vi "Sequencer UI - User Event - Inbound&Outbound (Solution).vi"(10 "Outbound User Events":T1, 11 "Inbound User Events":T2) -> ()   [LabVIEW 2019]
uses:
  typedefs/step.data--Cluster.ctl
  typedefs/step.IO.data--Cluster.ctl
  typedefs/IOType--Enum.ctl
  <userlib>/_OpenG.lib/file/file.llb/File Exists - Scalar__ogtk.vi
  <userlib>/_OpenG.lib/file/file.llb/Valid Path - Traditional__ogtk.vi
panel:
  out "timer value":u32
  out "Seq. Aborted?":bool
  out "Seq. Loaded?":bool
  out "Seq. Running?":bool
  out "AO Chart":cluster{"[0]":dbl, "[1]":dbl}(graph)
  out "Running Step ID":string caption="Step ID"
  out "States History":string caption="Last State"
  out "Sequence MCL Ref":i32(listbox) caption="Sequence"
  in  "Abort Sequence":bool
  in  "Run Sequence":bool
  in  "Load Sequence":bool
  in  "Exit":bool
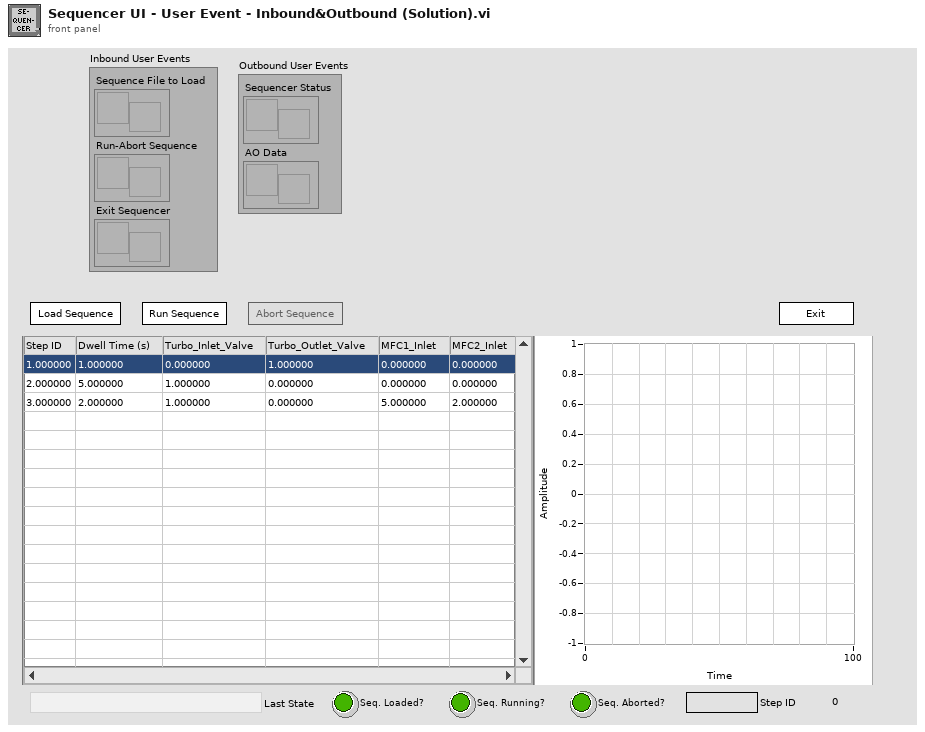
[diagram p1: front panel]
types:
  T1 = cluster{"Sequencer Status":refnum<user-event>, "AO Data":refnum<user-event>}
  T2 = cluster{"Sequence File to Load":refnum<user-event>, "Run-Abort Sequence":refnum<user-event>, "Exit Sequencer":refnum<user-event>}
  T3 = enum32{"invalid app kind", "Development System", "Run Time System", "Student Edition", "Embedded LabVIEW", "Evaluation", "Custom"}
  T4 = enum32{"Invalid", "Standard", "Closed", "Hidden", "Minimized", "Maximized"}
  T5 = enum8{"Enabled", "Disabled", "Disabled and Grayed Out"}
  T6 = typedef "step.data--Cluster.ctl" = cluster{"Step ID":string, "Dwell Time(s)":dbl, "Recipe Step":T7[]}
  T7 = typedef "step.IO.data--Cluster.ctl" = cluster{"IO Name":string, "IO Type":T8, "IO Value":variant}
  T8 = typedef "IOType--Enum.ctl" = enum16{"<Undefined>", "DO", "DI", "AO", "AI"}
  T9 = cluster{"Core":cluster{"Current VI Reference":refnum<vi>, "Close Panel on Exit?":bool}, "Seq. Loaded?":bool, "Sequence file path":path, "Sequence Data [ ]":T6[], "Sequence MCL Ref":refnum<vi>, "DO Data [ ]":cluster{"DO Name":string, "DO Value":variant}[], "AO Data [ ]":cluster{"AO Name":string, "AO Value":variant}[], "Running Step #":i32, "Seq. Running?":bool, "Seq. Aborted?":bool, "Inbound User Events":cluster{"Sequence File to Load":refnum<user-event>, "Run-Abort Sequence":refnum<user-event>, "Exit Sequencer":refnum<user-event>}, "Outbound User Events":cluster{"Sequencer Status":refnum<user-event>, "AO Data":refnum<user-event>}}
  T10 = cluster{"Current VI Reference":refnum<vi>, "Close Panel on Exit?":bool}
  T11 = cluster{"Seq. Loaded?":bool, "Seq. Running?":bool, "Seq. Aborted?":bool}
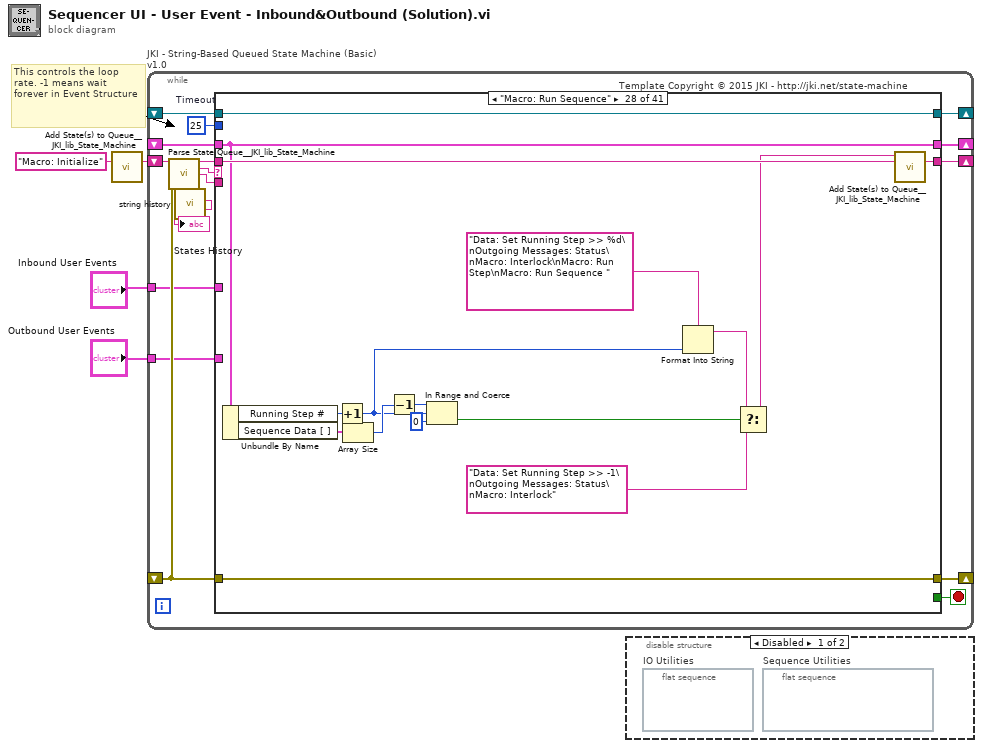
[diagram p0: block diagram]
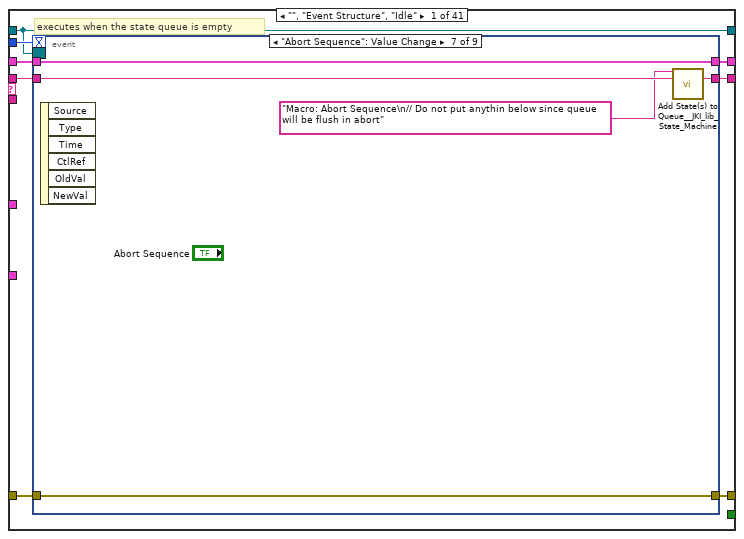
[diagram p3: hidden frame]
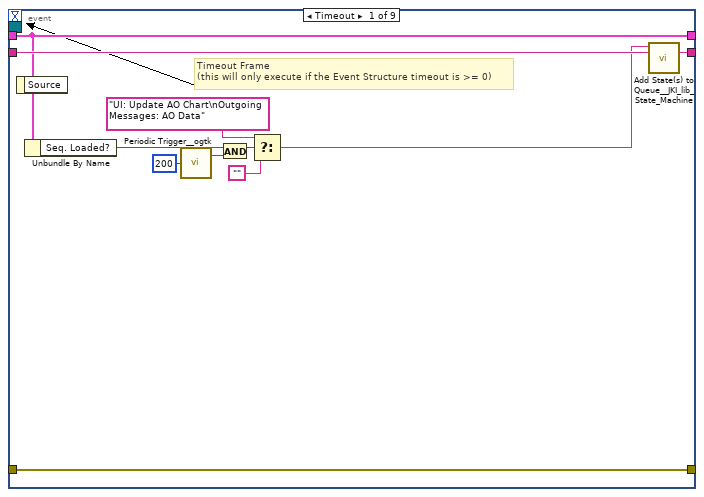
[diagram p4: hidden frame]
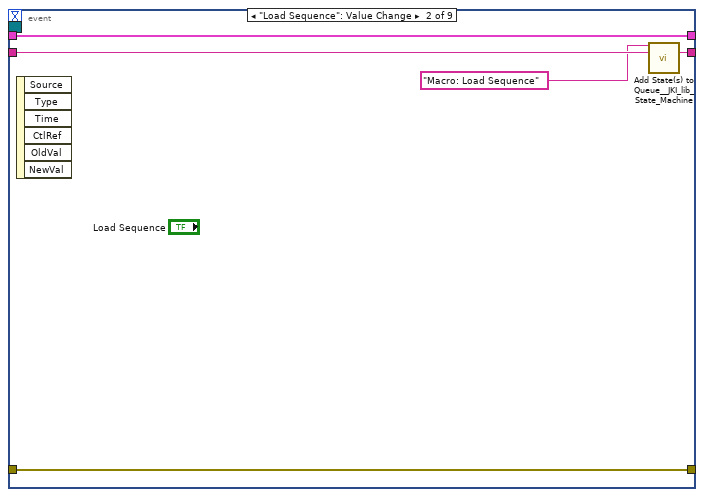
[diagram p5: hidden frame]
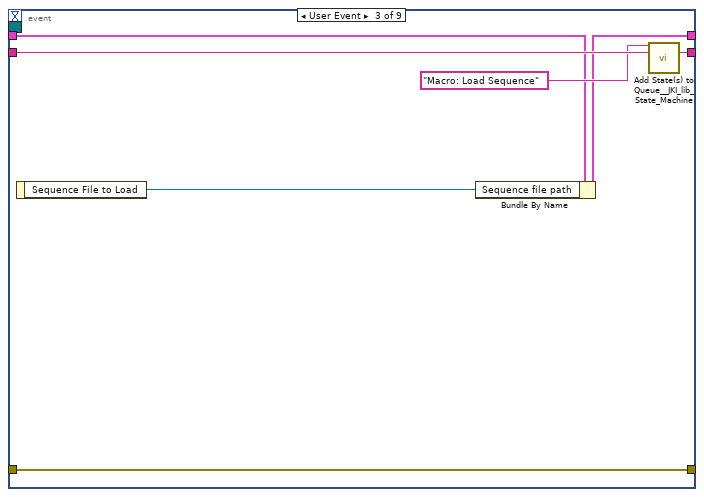
[diagram p6: hidden frame]
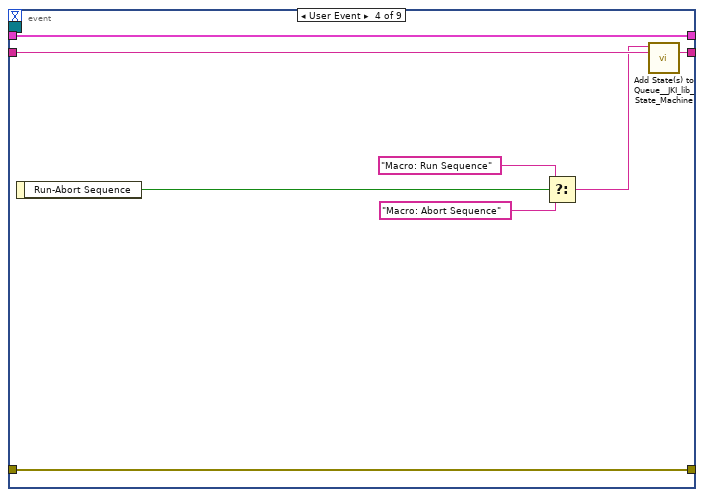
[diagram p7: hidden frame]
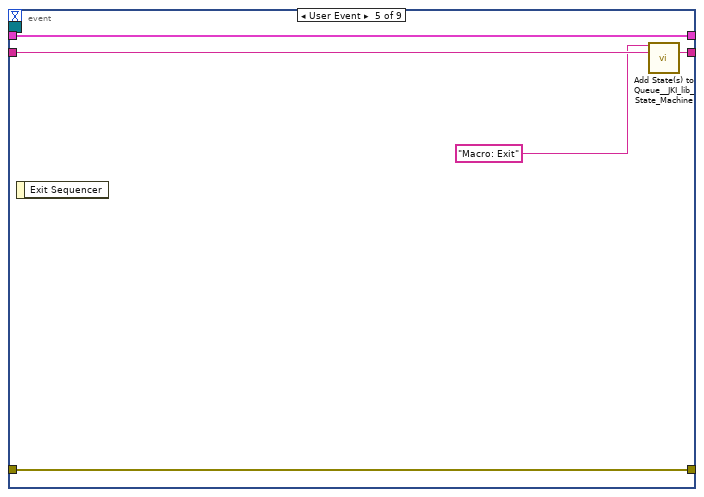
[diagram p8: hidden frame]
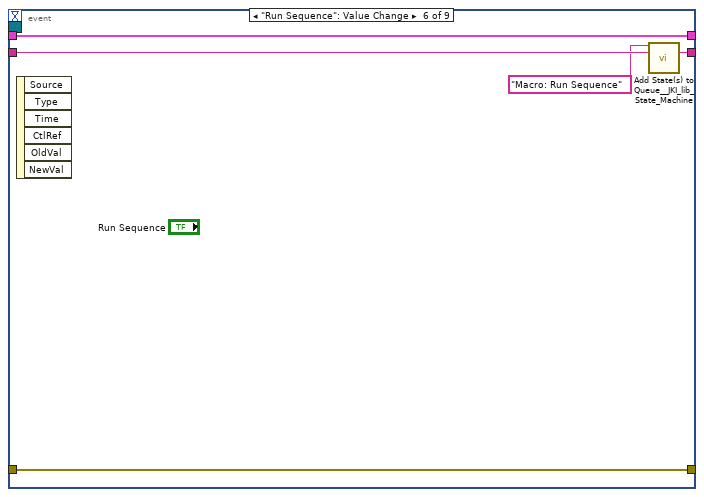
[diagram p9: hidden frame]
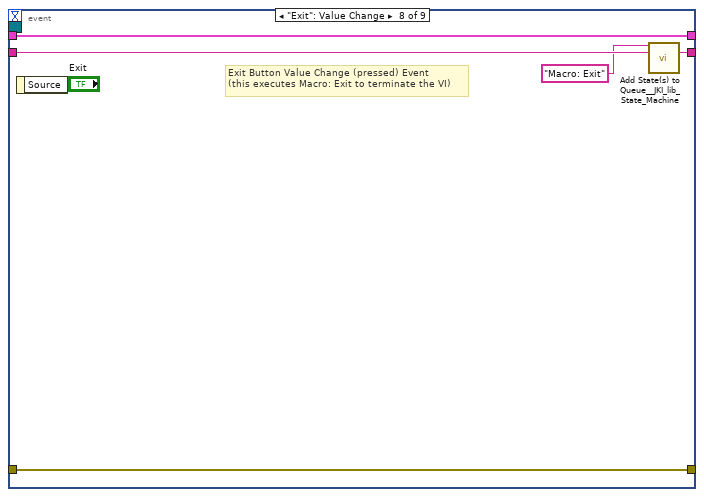
[diagram p10: hidden frame]
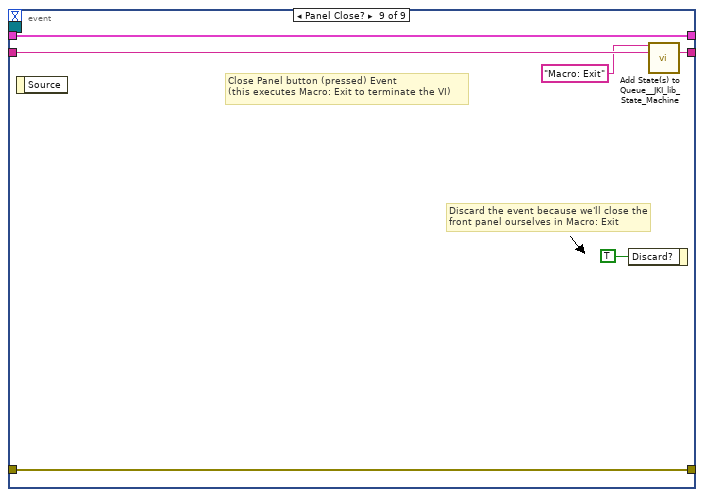
[diagram p11: hidden frame]
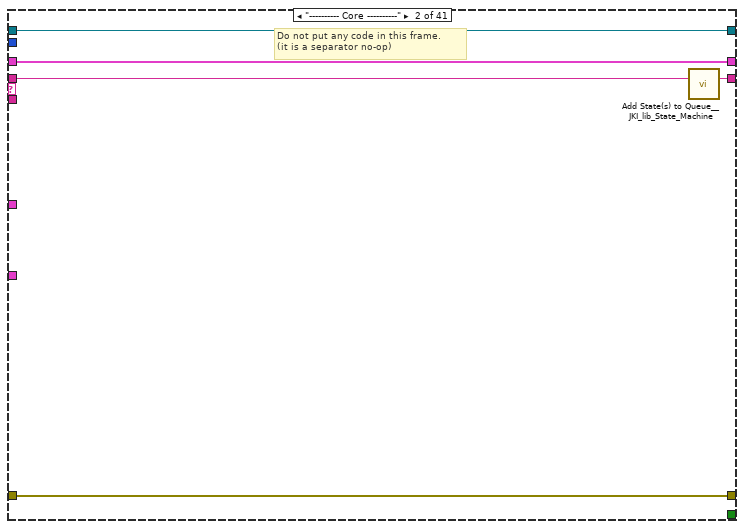
[diagram p12: hidden frame]
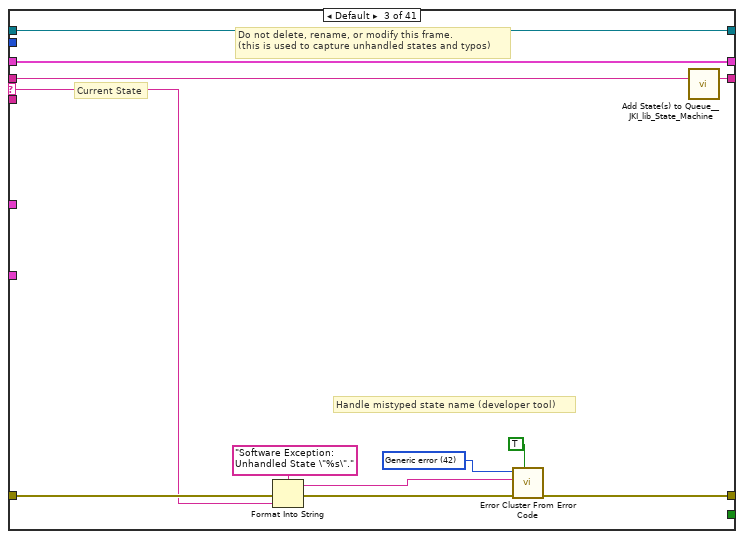
[diagram p13: hidden frame]
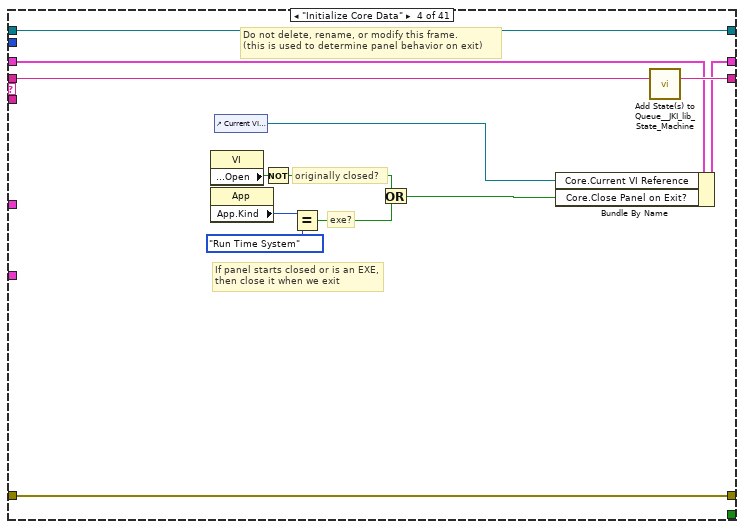
[diagram p14: hidden frame]
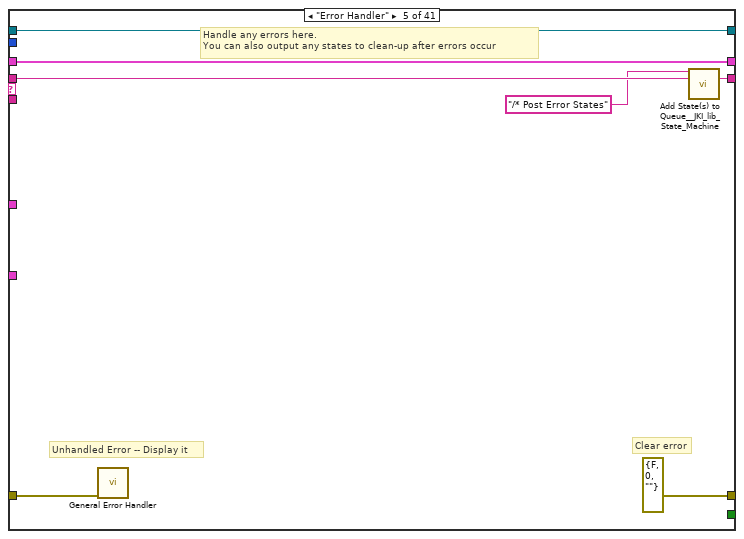
[diagram p15: hidden frame]
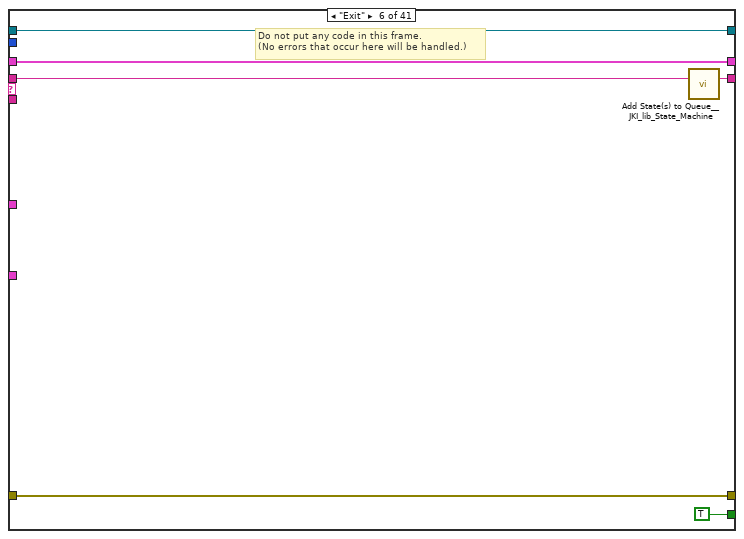
[diagram p16: hidden frame]
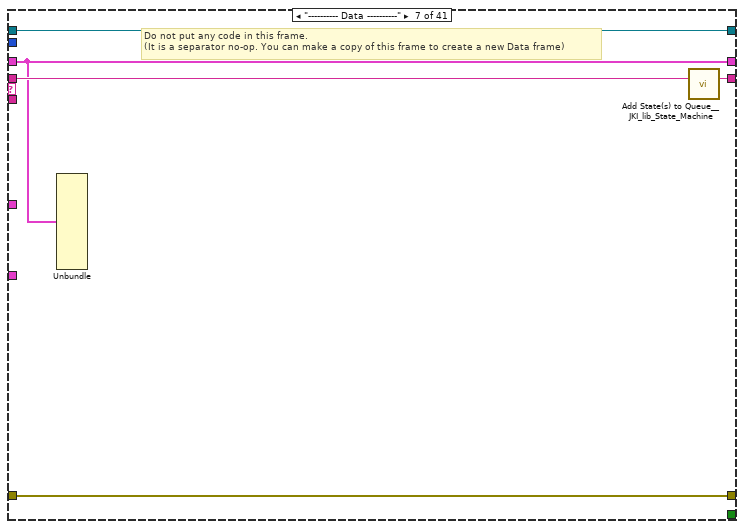
[diagram p17: hidden frame]
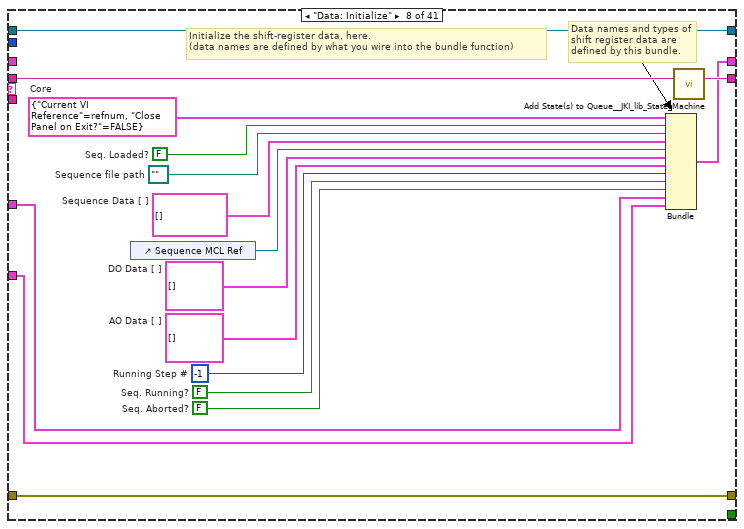
[diagram p18: hidden frame]
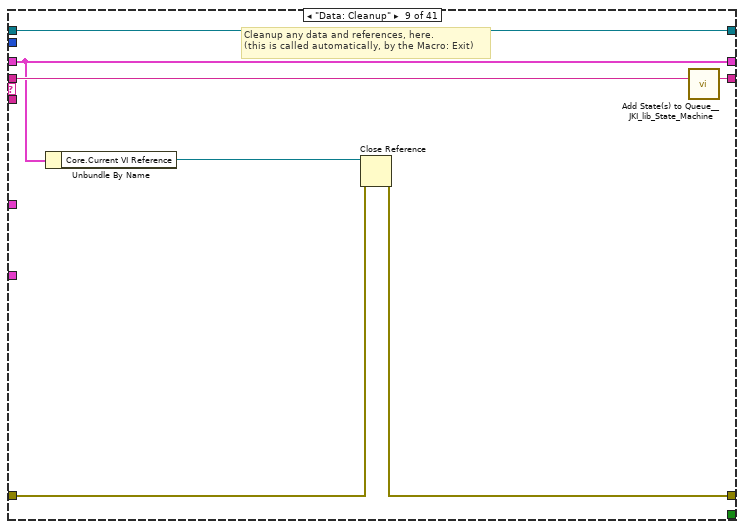
[diagram p19: hidden frame]
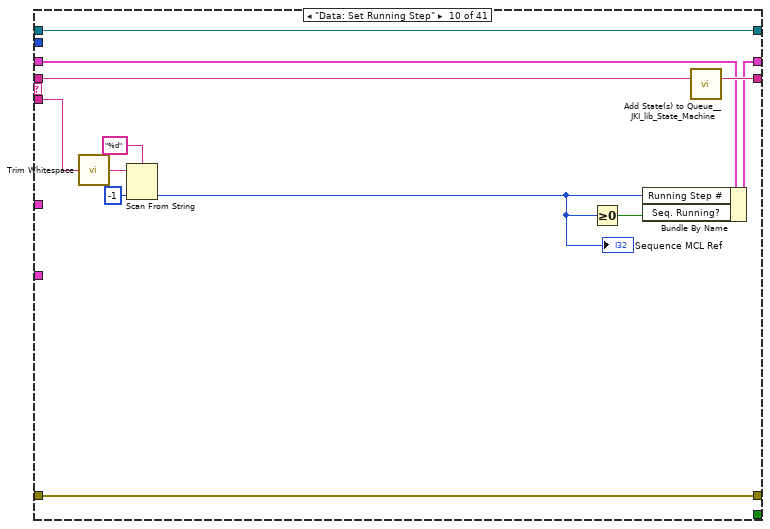
[diagram p20: hidden frame]
diagram:
  # "This controls the loop rate. -1 means wait forever in Event Structure"
  n1 = call <vilib>:"Add State(s) to Queue__JKI_lib_State_Machine.vi"("State(s) in (\"\")"="Macro: Initialize") -> ("States Out"=w4:string)  [unwired: 14 in]
  n2 = while "JKI - String-Based Queued State Machine (Basic) v1.0" {
    shift-right: [w14] -> _
    shift-left: _ -> [w13]
    shift-right: [w17] -> _
    shift-left: _ -> [w11]
    shift-right: [w16] -> _
    shift-left: w4 -> [w18]
    tunnel: "Inbound User Events" -> [w8]
    shift-right: [w7] -> _
    shift-left: _ -> [w6]
    tunnel: "Outbound User Events" -> [w5]
    stop <- w15 stop-if-true
    w12 = 25  # Timeout
    # "Template Copyright © 2015 JKI - http://jki.net/state-machine"
    n3 = call <vilib>:"Parse State Queue__JKI_lib_State_Machine.vi"("State Queue"=w18, "Error In (no error)"=w11) -> ("Remaining States"=w20:string, "Current State"=w10:string, "Arguments"=w19:string)  [unwired: 11 in]
    n4 = call "string history.vi"("State Queue"=w10) -> ("State Queue history (last on top)"=→"States History":string)  [unwired: 10 in]
    n5 = case shown="\"Macro: Run Sequence\"" w10 {
      selector: w10 -> [_ _ w92 _ _ _ _ _ _ _ _ _ _ _ _ _ _ _ _ _ _ _ _ _ _ _ _ _ _ _ _ _ _ _ _ _ _ _ _ _ _]
      tunnel: w20 -> [w28 w90 w96 w115 w122 w128 w133 w150 w157 w169 w180 w191 w196 w203 w209 w214 w225 w232 w244 w274 w286 w298 w321 w326 w332 w338 w344 w360 w366 _ w382 w387 w394 w401 w420 w425 w438 w456 w461 w474 w494]
      tunnel: w19 -> [_ _ _ _ _ _ _ _ _ w164 w172 w183 _ _ _ _ _ w227 w238 _ _ _ _ _ _ _ _ _ _ _ _ _ _ _ _ _ _ _ _ _ _]
      tunnel: w13 -> [w26 w87 w94 w106 w119 w126 w130 _ w152 w167 w178 w189 w193 w199 w207 w211 w223 w230 w240 w272 w283 w288 w319 w323 w329 w335 w341 w357 w363 w370 w379 w384 w390 w399 w414 w422 w435 w451 w458 w471 w483]
      tunnel: [w25 w88 w98 w112 errorcluster {"status"=FALSE, "code"=0, "source"=""} ("error out") w125 w131 w147 w153 w166 w177 w188 w194 w200 w204 w212 w218 w228 w241 w269 w284 w296 w313 w324 w330 w336 w342 w358 w364 w369 w380 w385 w391 w396 w413 w423 w429 w452 w459 w466 w491] -> w17
      tunnel: w11 -> [w24 w88 w97 w112 w118 w125 w131 w147 w154 w166 w177 w188 w194 w197 w205 w212 w219 w229 w242 w270 w284 w296 w314 w324 w330 w336 w342 w358 w364 w369 w380 w385 w392 w397 w413 w423 w430 w453 w459 w465 w480]
      tunnel: [w27 w89 w95 w114 w121 w127 w132 w149 w156 w168 w179 w190 w195 w202 w208 w213 w224 w231 w243 w273 w285 w297 w320 w325 w331 w337 w343 w359 w365 w371 w381 w386 w393 w400 w419 w424 w437 w455 w460 w473 w493] -> w16
      tunnel: [_ _ _ _ _ TRUE _ _ _ _ _ _ _ _ _ _ _ _ _ _ _ _ _ _ _ _ _ _ _ _ _ _ _ _ _ _ _ _ _ _ _] -> w15
      tunnel: [w23 w87 w94 w113 w119 w126 w130 w148 w152 w165 w176 w187 w193 w199 w207 w211 w223 w230 w240 w272 w283 w288 w319 w323 w329 w335 w341 w357 w363 w370 w379 w384 w390 w399 w414 w422 w436 w454 w458 w471 w483] -> w14
      tunnel: w12 -> [w22 _ _ _ _ _ _ _ _ _ _ _ _ _ _ _ _ _ _ _ _ _ _ _ _ _ _ _ _ _ _ _ _ _ _ _ _ _ _ _ _]
      tunnel: w8 -> [_ _ _ _ _ _ _ w136 _ _ _ _ _ _ _ _ _ _ _ _ _ _ _ _ _ _ _ _ _ _ _ _ _ _ _ _ _ _ _ _ _]
      tunnel: [w21 w86 w91 w103 w116 w123 w129 w135 w151 w158 w170 w181 w192 w201 w206 w210 w215 w226 w237 w267 w275 w287 w311 w322 w327 w333 w339 w345 w361 w367 w372 w383 w388 w395 w402 w421 w426 w446 w457 w472 w492] -> w7
      tunnel: w6 -> [w21 w86 w91 w103 w116 w123 w129 w135 w151 w158 w170 w181 w192 _ w206 w210 w215 w226 w237 w267 w275 w287 w311 w322 w327 w333 w339 w345 w361 w367 w372 w383 w388 w395 w402 w421 w426 w446 w457 w472 w492]
      tunnel: w5 -> [_ _ _ _ _ _ _ w134 _ _ _ _ _ _ _ _ _ _ _ _ _ _ _ _ _ _ _ _ _ _ _ _ _ _ _ _ _ _ _ _ _]
      frame "", "Event Structure", "Idle" {
        # "executes when the state queue is empty"
        n6 = event shown="[6] \"Abort Sequence\": Value Change" {
          selector: w21 -> [_ _ _ _ _ _ _ _ _]
          dyn-events: _ -> [_ _ _ _ _ _ _ _ _]
          timeout: w22 -> [_ _ _ _ _ _ _ _ _]
          tunnel: w28 -> [w39 w44 w51 w59 w64 w69 w74 w79 w85]
          tunnel: [w38 w43 w50 w58 w63 w68 w73 w78 w84] -> w27
          tunnel: w26 -> [w30 w41 w46 w56 w61 w66 w71 w76 w82]
          tunnel: [w37 w42 w49 w57 w62 w67 w72 w77 w83] -> w25
          tunnel: w24 -> [w37 w42 w49 w57 w62 w67 w72 w77 w83]
          tunnel: [w30 w41 w47 w56 w61 w66 w71 w76 w82] -> w23
          event Timeout {
            # "Timeout Frame\n(this will only execute if the Event Structure timeout is >= 0)"
            n7 = event-data() -> ()  [unwired: 1 in, 1 out]
            n8 = Unbundle By Name(w30) -> ("Seq. Loaded?"=w32:bool)
            n9 = call <userlib>:"Periodic Trigger__ogtk.vi"("time (ms)"=u32 200) -> ("Triggered"=w36:bool)  [unwired: 12 in, 2 out]
            n10 = And(x=w32, y=w36) -> (x .and. y?=w35:bool)
            n11 = Select(t="UI: Update AO Chart\nOutgoing Messages: AO Data", s=w35, f="") -> (s? t:f=w29:string)
            n12 = call <vilib>:"Add State(s) to Queue__JKI_lib_State_Machine.vi"("State(s) in Front (\"\")"=w29, "State(s) in (\"\")"=w39) -> ("States Out"=w38:string)  [unwired: 13 in]
          }
          event "Load Sequence": Value Change {
            n13 = event-data() -> ()  [unwired: 1 in, 6 out]
            n14 = call <vilib>:"Add State(s) to Queue__JKI_lib_State_Machine.vi"("State(s) in Front (\"\")"="Macro: Load Sequence", "State(s) in (\"\")"=w44) -> ("States Out"=w43:string)  [unwired: 13 in]
          }
          event User Event {
            n15 = event-data() -> ("Sequence File to Load"=w45:path)  [unwired: 1 in]
            n16 = Bundle By Name(cluster=w46, "Sequence file path"=w45) -> (w47:T9)
            n17 = call <vilib>:"Add State(s) to Queue__JKI_lib_State_Machine.vi"("State(s) in Front (\"\")"="Macro: Load Sequence", "State(s) in (\"\")"=w51) -> ("States Out"=w50:string)  [unwired: 13 in]
          }
          event User Event {
            n18 = event-data() -> ("Run-Abort Sequence"=w53:bool)  [unwired: 1 in]
            n19 = Select(t="Macro: Run Sequence", s=w53, f="Macro: Abort Sequence") -> (s? t:f=w52:string)
            n20 = call <vilib>:"Add State(s) to Queue__JKI_lib_State_Machine.vi"("State(s) in Front (\"\")"=w52, "State(s) in (\"\")"=w59) -> ("States Out"=w58:string)  [unwired: 13 in]
          }
          event User Event {
            n21 = event-data() -> ()  [unwired: 1 in, 1 out]
            n22 = call <vilib>:"Add State(s) to Queue__JKI_lib_State_Machine.vi"("State(s) in Front (\"\")"="Macro: Exit", "State(s) in (\"\")"=w64) -> ("States Out"=w63:string)  [unwired: 13 in]
          }
          event "Run Sequence": Value Change {
            n23 = event-data() -> ()  [unwired: 1 in, 6 out]
            n24 = call <vilib>:"Add State(s) to Queue__JKI_lib_State_Machine.vi"("State(s) in Front (\"\")"="Macro: Run Sequence", "State(s) in (\"\")"=w69) -> ("States Out"=w68:string)  [unwired: 13 in]
          }
          event "Abort Sequence": Value Change {
            n25 = event-data() -> ()  [unwired: 1 in, 6 out]
            n26 = call <vilib>:"Add State(s) to Queue__JKI_lib_State_Machine.vi"("State(s) in Front (\"\")"="Macro: Abort Sequence\n// Do not put anythin below since queue will be flush in abort", "State(s) in (\"\")"=w74) -> ("States Out"=w73:string)  [unwired: 13 in]
          }
          event "Exit": Value Change {
            # "Exit Button Value Change (pressed) Event\n(this executes Macro: Exit to terminate the VI)"
            n27 = event-data() -> ()  [unwired: 1 in, 1 out]
            n28 = call <vilib>:"Add State(s) to Queue__JKI_lib_State_Machine.vi"("State(s) in Front (\"\")"="Macro: Exit", "State(s) in (\"\")"=w79) -> ("States Out"=w78:string)  [unwired: 13 in]
          }
          event Panel Close? {
            # "Discard the event because we'll close the front panel ourselves in Macro: Exit"
            # "Close Panel button (pressed) Event\n(this executes Macro: Exit to terminate the VI)"
            n29 = event-data() -> ()  [unwired: 1 in, 1 out]
            n30 = event-data("Discard?"=TRUE) -> ()  [unwired: 1 in, 1 out]
            n31 = call <vilib>:"Add State(s) to Queue__JKI_lib_State_Machine.vi"("State(s) in Front (\"\")"="Macro: Exit", "State(s) in (\"\")"=w85) -> ("States Out"=w84:string)  [unwired: 13 in]
          }
        }
      }
      frame "---------- Core ----------" {
        # "Do not put any code in this frame.\n(it is a separator no-op)"
        n32 = call <vilib>:"Add State(s) to Queue__JKI_lib_State_Machine.vi"("State(s) in (\"\")"=w90) -> ("States Out"=w89:string)  [unwired: 14 in]
      }
      frame Default {
        w101 = 42 items=["No error", "Argument error", "Memory is full", "Out of zone", "End of file", "File already open", "Generic file I/O error", "File not found", "File permission error", "Disk is full", "Duplicate path", "Too many files open", "System feature not enabled", "Resource file not found", "Cannot add resource", "Resource not found", "Image not found", "Image memory error", "Pen does not exist", "Config type invalid", "Config token not found", "Config parse error", "Config memory error", "Bad external code format", "Bad external code offset", "External code not present", "Null window", "Destroy window error", "Null menu", "Print aborted", "Bad print record", "Print driver error", "Windows error during printing", "Memory error during printing", "Print dialog error", "Generic print error", "Invalid device refnum", "Device not found", "Device parameter error", "Device unit error", "Cannot open device", "Device call aborted", "Generic error", "Cancelled by user", "Object ID too low", "Object ID too high", "Object not in heap", "Unknown heap", "Unknown object (invalid DefProc)", "Unknown object (DefProc not in table)", "Message out of range", "Invalid (null) method", "Unknown message", "Manager call not supported", "Bad address", "Network operation in progress", "Network operation timed out", "Connection is busy", "Network attribute not supported", "Network error", "Address in use", "System out of memory", "Connection aborted", "Connection refused", "Not connected", "Already connected", "Connection closed", "Initialization error (interapplication manager)", "Bad occurrence", "Wait on unbound occurrence handler", "Occurrence queue overflow", "Datalog type conflict", "Unused", "Unrecognized type (interapplication manager)", "Memory corrupt", "Failed to make temporary DLL", "Old CIN version", "Drag socket not found", "Failed to load drop-object", "Failed to register OLE object", "Failed to release OLE object", "Format specifier type mismatch", "Unknown format specifier", "Too few format specifiers", "Too many format specifiers", "Scan failed", "Newer CIN version", "Error converting to variant", "Runtime menu error", "Password tampered", "Variant attribute not found", "Incompatible variant data type", "Event data is not available", "Event Store is not present", "Occurrence is not found", "Event Queue is not created", "Event info is not available", "Refnum passed is NULL", "Error retrieving Class GUID", "Error retrieving CoClass GUID", "Error retrieving TypeLib GUID.", "Bad built application magic bytes.", "Specific driver is different from the specific driver associated with the Logical Name.", "There is no session opened to the class driver.", "Max Error", "MAX - Error with config objects", "MAX - Error loading configuration", "MAX - Group not supported"]
        # "Current State"
        # "Do not delete, rename, or modify this frame.\n(this is used to capture unhandled states and typos)"
        # "Handle mistyped state name (developer tool)"
        n33 = Format Into String(format string="Software Exception: Unhandled State \"%s\"." ("message"), error in=w97, w92) -> (resulting string=w100:string, error out=w99:errorcluster)  [unwired: 1 in]
        n34 = call <vilib>:"Error Cluster From Error Code.vi"("show call chain? (False)"=TRUE, "error in (no error)"=w99, "error message (\"\")"=w100, "error code (0)"=w101) -> ("error out"=w98:errorcluster)  [unwired: 5 in]
        n35 = call <vilib>:"Add State(s) to Queue__JKI_lib_State_Machine.vi"("State(s) in (\"\")"=w96) -> ("States Out"=w95:string)  [unwired: 14 in]
      }
      frame "Initialize Core Data" {
        # "Do not delete, rename, or modify this frame.\n(this is used to determine panel behavior on exit)"
        # "originally closed?"
        # "exe?"
        # "If panel starts closed or is an EXE, then close it when we exit"
        n36 = property class="VI"() -> ("Front Panel.Open"=w111:bool)  [unwired: 2 in, 2 out]
        n37 = property class="App"() -> ("App.Kind"=w110:T3)  [unwired: 2 in, 2 out]
        n38 = control-ref of="Current VI Reference"() -> (w104:refnum<vi>)
        n39 = Not(x=w111) -> (.not. x?=w108:bool)
        n40 = Equal?(x=w110, y=T3."Run Time System" ("Application:Kind")) -> (x = y?=w107:bool)
        n41 = Or(x=w108, y=w107) -> (x .or. y?=w105:bool)
        n42 = Bundle By Name(cluster=w106, "Core.Current VI Reference"=w104, "Core.Close Panel on Exit?"=w105) -> (w113:T9)
        n43 = call <vilib>:"Add State(s) to Queue__JKI_lib_State_Machine.vi"("State(s) in (\"\")"=w115) -> ("States Out"=w114:string)  [unwired: 14 in]
      }
      frame "Error Handler" {
        # "Unhandled Error -- Display it"
        # "Handle any errors here.\nYou can also output any states to clean-up after errors occur"
        # "Clear error"
        n44 = call <vilib>:"General Error Handler.vi"("error in (no error)"=w118) -> ()  [unwired: 10 in, 5 out]
        n45 = call <vilib>:"Add State(s) to Queue__JKI_lib_State_Machine.vi"("State(s) in Front (\"\")"="/* Post Error States", "State(s) in (\"\")"=w122) -> ("States Out"=w121:string)  [unwired: 13 in]
      }
      frame "Exit" {
        # "Do not put any code in this frame.\n(No errors that occur here will be handled.)"
        n46 = call <vilib>:"Add State(s) to Queue__JKI_lib_State_Machine.vi"("State(s) in (\"\")"=w128) -> ("States Out"=w127:string)  [unwired: 14 in]
      }
      frame "---------- Data ----------" {
        # "Do not put any code in this frame.\n(It is a separator no-op. You can make a copy of this frame to create a new Data frame)"
        n47 = Unbundle(w130) -> ()  [unwired: 12 out]
        n48 = call <vilib>:"Add State(s) to Queue__JKI_lib_State_Machine.vi"("State(s) in (\"\")"=w133) -> ("States Out"=w132:string)  [unwired: 14 in]
      }
      frame "Data: Initialize" {
        w137 = path ""  # Sequence file path
        w138 = FALSE  # Seq. Aborted?
        w139 = FALSE  # Seq. Running?
        w140 = -1  # Running Step #
        w141 = cluster{"AO Name":string, "AO Value":variant}[] []  # AO Data [ ]
        w142 = cluster{"DO Name":string, "DO Value":variant}[] []  # DO Data [ ]
        w144 = T6[] []  # Sequence Data [ ]
        w145 = T10 {"Current VI Reference"=refnum, "Close Panel on Exit?"=FALSE}  # Core
        w146 = FALSE  # Seq. Loaded?
        # "Data names and types of shift register data are defined by this bundle."
        # "Initialize the shift-register data, here.\n(data names are defined by what you wire into the bundle function)"
        n49 = control-ref of="Sequence MCL Ref"() -> (w143:refnum<vi>)
        n50 = Bundle("Core"=w145, "Seq. Loaded?"=w146, "Sequence file path"=w137, "Sequence Data [ ]"=w144, "Sequence MCL Ref"=w143, "DO Data [ ]"=w142, "AO Data [ ]"=w141, "Running Step #"=w140, "Seq. Running?"=w139, "Seq. Aborted?"=w138, "Inbound User Events"=w136, "Outbound User Events"=w134) -> (w148:T9)  [unwired: 1 in]
        n51 = call <vilib>:"Add State(s) to Queue__JKI_lib_State_Machine.vi"("State(s) in (\"\")"=w150) -> ("States Out"=w149:string)  [unwired: 14 in]
      }
      frame "Data: Cleanup" {
        # "Cleanup any data and references, here.\n(this is called automatically, by the Macro: Exit)"
        n52 = Unbundle By Name(w152) -> ("Core.Current VI Reference"=w155:refnum<vi>)
        n53 = Close Reference(reference=w155, error in (no error)=w154) -> (error out=w153:errorcluster)
        n54 = call <vilib>:"Add State(s) to Queue__JKI_lib_State_Machine.vi"("State(s) in (\"\")"=w157) -> ("States Out"=w156:string)  [unwired: 14 in]
      }
      frame "Data: Set Running Step" {
        n55 = call <vilib>:"Trim Whitespace.vi"("string"=w164) -> ("trimmed string"=w163:string)  [unwired: 1 in]
        n56 = Scan From String(format string="%d", input string=w163, default 1=-1 ("default value 1")) -> (output 1=w159:i32)  [unwired: 2 in, 3 out]
        "Sequence MCL Ref" <- w159
        n57 = Greater Or Equal To 0?(x=w159) -> (x >= 0?=w160:bool)
        n58 = Bundle By Name(cluster=w167, "Running Step #"=w159, "Seq. Running?"=w160) -> (w165:T9)
        n59 = call <vilib>:"Add State(s) to Queue__JKI_lib_State_Machine.vi"("State(s) in (\"\")"=w169) -> ("States Out"=w168:string)  [unwired: 14 in]
      }
      frame "Data: Set Seq. Loaded Flag" {
        n60 = call <vilib>:"Trim Whitespace.vi"("string"=w172) -> ("trimmed string"=w175:string)  [unwired: 1 in]
        n61 = To Upper Case(1:w175) -> (0:w174:string)
        n62 = Equal?(x=w174, y="TRUE") -> (x = y?=w171:bool)
        n63 = Bundle By Name(cluster=w178, "Seq. Loaded?"=w171) -> (w176:T9)
        n64 = call <vilib>:"Add State(s) to Queue__JKI_lib_State_Machine.vi"("State(s) in (\"\")"=w180) -> ("States Out"=w179:string)  [unwired: 14 in]
      }
      frame "Data: Set Seq. Aborted Flag" {
        n65 = call <vilib>:"Trim Whitespace.vi"("string"=w183) -> ("trimmed string"=w186:string)  [unwired: 1 in]
        n66 = To Upper Case(1:w186) -> (0:w185:string)
        n67 = Equal?(x=w185, y="TRUE") -> (x = y?=w182:bool)
        n68 = Bundle By Name(cluster=w189, "Seq. Aborted?"=w182) -> (w187:T9)
        n69 = call <vilib>:"Add State(s) to Queue__JKI_lib_State_Machine.vi"("State(s) in (\"\")"=w191) -> ("States Out"=w190:string)  [unwired: 14 in]
      }
      frame "---------- Events ----------" {
        # "Do not put any code in this frame.\n(It is a separator no-op. You can make a copy of this frame to create a new UI frame)"
        n70 = call <vilib>:"Add State(s) to Queue__JKI_lib_State_Machine.vi"("State(s) in (\"\")"=w196) -> ("States Out"=w195:string)  [unwired: 14 in]
      }
      frame "Events: Register" {
        n71 = Unbundle By Name(w199) -> ("Inbound User Events"=w198:T2)
        n72 = register-events(error in=w197, w198) -> (reference out=w201:refnum<event-registration>, error out=w200:errorcluster)  [unwired: 1 in]
        n73 = call <vilib>:"Add State(s) to Queue__JKI_lib_State_Machine.vi"("State(s) in (\"\")"=w203) -> ("States Out"=w202:string)  [unwired: 14 in]
      }
      frame "Events: Unregister" {
        n74 = Unregister For Events(event registration refnum=w206, error in=w205) -> (error out=w204:errorcluster)
        n75 = call <vilib>:"Add State(s) to Queue__JKI_lib_State_Machine.vi"("State(s) in (\"\")"=w209) -> ("States Out"=w208:string)  [unwired: 14 in]
      }
      frame "---------- UI ----------" {
        # "Do not put any code in this frame.\n(It is a separator no-op. You can make a copy of this frame to create a new UI frame)"
        n76 = call <vilib>:"Add State(s) to Queue__JKI_lib_State_Machine.vi"("State(s) in (\"\")"=w214) -> ("States Out"=w213:string)  [unwired: 14 in]
      }
      frame "UI: Initialize" {
        # "Initialize (empty) the multicolum list box"
        n77 = Unbundle By Name(w223) -> ("Running Step #"=w217:i32, "Sequence MCL Ref"=w222:refnum<vi>)
        n78 = property class="MCListbox (strict)"(reference=w222, error in=w219, "ItemNames"=string[][] [] ("Item Names"), "ColHdrString"=string[] [] ("Column Header Strings[]")) -> (error out=w218:errorcluster)  [unwired: 1 out]
        n79 = local write "Sequence MCL Ref"(w217) -> ()
        n80 = property on="AO Chart" class="WFChart (strict)"("History Data"=cluster{"[0]":dbl, "[1]":dbl}[] []) -> ()  [unwired: 2 in, 2 out]
        n81 = call <vilib>:"Add State(s) to Queue__JKI_lib_State_Machine.vi"("State(s) in (\"\")"=w225) -> ("States Out"=w224:string)  [unwired: 14 in]
      }
      frame "UI: Cursor Set" {
        # "Argument"
        # "Set and Unset Cursor Busy.\n(Usage: \"UI: Cursor Set >> Busy|Idle\")"
        n82 = case shown="\"Idle\", Default" w227 {
          tunnel: w229 -> [w234 w236]
          tunnel: [w233 w235] -> w228
          frame "Idle", Default {
            n83 = call <vilib>:"Unset Busy.vi"("error in (no error)"=w234) -> ("error out"=w233:errorcluster)  [unwired: 10 in]
          }
          frame "Busy" {
            n84 = call <vilib>:"Set Busy.vi"("error in (no error)"=w236) -> ("error out"=w235:errorcluster)  [unwired: 9 in, 1 out]
          }
        }
        n85 = call <vilib>:"Add State(s) to Queue__JKI_lib_State_Machine.vi"("State(s) in (\"\")"=w232) -> ("States Out"=w231:string)  [unwired: 14 in]
      }
      frame "UI: Front Panel State" {
        # "Argument"
        # "Set Front Panel Open or Closed\n(Usage: \"UI: Front Panel State >> Open|Close\")"
        n86 = Unbundle By Name(w240) -> ("Core.Current VI Reference"=w239:refnum<vi>)
        n87 = case shown="\"Open\", Default" w238 {
          tunnel: w242 -> [w248 w261]
          tunnel: [w250 w262] -> w241
          tunnel: w239 -> [w249 w259]
          frame "Open", Default {
            n88 = property class="VI"(reference=w249, error in=w248) -> (reference out=w246:refnum<vi>, error out=w247:errorcluster, "Front Panel.Open"=w245:bool)
            n89 = case shown="False" w245 {
              tunnel: [w253 w256] -> w250
              tunnel: w247 -> [w252 w256]
              tunnel: w246 -> [w251 _]
              frame False {
                n90 = invoke class="VI" method="FP.Open"(reference=w251, error in=w252, "Activate"=TRUE, "State"=T4."Standard") -> (error out=w253:errorcluster)  [unwired: 1 in, 4 out]
              }
              frame True {
              }
            }
          }
          frame "Close" {
            n91 = property class="VI"(reference=w259, error in=w261) -> (reference out=w258:refnum<vi>, error out=w260:errorcluster, "Front Panel.Open"=w257:bool)
            n92 = case shown="True" w257 {
              tunnel: [w263 w266] -> w262
              tunnel: w260 -> [w263 w265]
              tunnel: w258 -> [_ w264]
              frame False {
              }
              frame True {
                n93 = invoke class="VI" method="FP.Close"(reference=w264, error in=w265) -> (error out=w266:errorcluster)  [unwired: 1 in, 2 out]
              }
            }
          }
        }
        n94 = call <vilib>:"Add State(s) to Queue__JKI_lib_State_Machine.vi"("State(s) in (\"\")"=w244) -> ("States Out"=w243:string)  [unwired: 14 in]
      }
      frame "UI: Update MCL" {
        # "Set Front Panel Open or Closed\n(Usage: \"UI: Front Panel State >> Open|Close\")"
        n95 = Unbundle By Name(w272) -> ("Sequence MCL Ref"=w271:refnum<vi>, "Sequence Data [ ]"=w268:T6[])
        n96 = call "Sequence.PopulateMCL.vi"("error in (no error)"=w270, "Sequence Data"=w268, "MCListbox Refnum"=w271) -> ("error out"=w269:errorcluster)  [unwired: 8 in]
        n97 = call <vilib>:"Add State(s) to Queue__JKI_lib_State_Machine.vi"("State(s) in (\"\")"=w274) -> ("States Out"=w273:string)  [unwired: 14 in]
      }
      frame "UI: Update Status" {
        # "Set Front Panel Open or Closed\n(Usage: \"UI: Front Panel State >> Open|Close\")"
        n98 = Unbundle By Name(w283) -> ("Seq. Loaded?"=→"Seq. Loaded?":bool, "Seq. Running?"=→"Seq. Running?":bool, "Seq. Aborted?"=→"Seq. Aborted?":bool)
        n99 = Unbundle By Name(w283) -> ("Sequence Data [ ]"=w281:T6[], "Running Step #"=w282:i32)
        n100 = Index Array(array=w281, index=w282) -> (element=w280:T6)
        n101 = Unbundle By Name(w280) -> ("Step ID"=→"Running Step ID":string)
        n102 = call <vilib>:"Add State(s) to Queue__JKI_lib_State_Machine.vi"("State(s) in (\"\")"=w286) -> ("States Out"=w285:string)  [unwired: 14 in]
      }
      frame "UI: Update Interlock" {
        # "Set Front Panel Open or Closed\n(Usage: \"UI: Front Panel State >> Open|Close\")"
        n103 = Unbundle By Name(w288) -> ("Seq. Loaded?"=w295:bool, "Seq. Running?"=w294:bool)
        n104 = case shown="True" w295 {
          tunnel: w294 -> [_ w306]
          tunnel: [w299 w302] -> w293
          tunnel: [w300 w303] -> w292
          tunnel: [w300 w301] -> w291
          tunnel: T5."Disabled and Grayed Out" ("Disabled") -> [w300 w305]
          tunnel: T5."Enabled" ("Disabled") -> [w299 w304]
          frame False {
          }
          frame True {
            n105 = case shown="False" w306 {
              tunnel: w305 -> [w308 w309]
              tunnel: w304 -> [w307 w310]
              tunnel: [w307 w309] -> w303
              tunnel: [w307 w309] -> w302
              tunnel: [w308 w310] -> w301
              frame False {
              }
              frame True {
              }
            }
          }
        }
        n106 = property on="Load Sequence" class="Bool"("DisabledEnum"=w293) -> ()  [unwired: 2 in, 2 out]
        n107 = property on="Run Sequence" class="Bool"("DisabledEnum"=w292) -> ()  [unwired: 2 in, 2 out]
        n108 = property on="Abort Sequence" class="Bool"("DisabledEnum"=w291) -> ()  [unwired: 2 in, 2 out]
        n109 = call <vilib>:"Add State(s) to Queue__JKI_lib_State_Machine.vi"("State(s) in (\"\")"=w298) -> ("States Out"=w297:string)  [unwired: 14 in]
      }
      frame "UI: Update AO Chart" {
        # "Set Front Panel Open or Closed\n(Usage: \"UI: Front Panel State >> Open|Close\")"
        n110 = Unbundle By Name(w319) -> ("Sequence Data [ ]"=w317:T6[], "Running Step #"=w316:i32)
        n111 = call "Sequence.GetStep.vi"("error in (no error)"=w314, "Step #"=w316, "Sequence Data"=w317) -> ("error out"=w315:errorcluster, "AO [ ]"=w318:cluster{"IO Name":string, "IO Value":variant}[])  [unwired: 6 in, 1 out]
        n112 = call "Graph.UpdateAOs.vi"("error in (no error)"=w315, "AO Data [ ]"=w318) -> ("error out"=w313:errorcluster, "Graph Data"=→"AO Chart":cluster{"[0]":dbl, "[1]":dbl})  [unwired: 8 in]
        n113 = call <vilib>:"Add State(s) to Queue__JKI_lib_State_Machine.vi"("State(s) in (\"\")"=w321) -> ("States Out"=w320:string)  [unwired: 14 in]
      }
      frame "---------- Macro ----------" {
        # "Do not put any code in this frame.\n(It is a separator no-op. You can make a copy of this frame to create a new Macro frame)"
        n114 = call <vilib>:"Add State(s) to Queue__JKI_lib_State_Machine.vi"("State(s) in (\"\")"=w326) -> ("States Out"=w325:string)  [unwired: 14 in]
      }
      frame "Macro: Initialize" {
        # "Initialization Macro\n(This is called once, when the VI starts)"
        n115 = call <vilib>:"Add State(s) to Queue__JKI_lib_State_Machine.vi"("State(s) in Front (\"\")"="Data: Initialize\nInitialize Core Data\nEvents: Register\nUI: Initialize\nUI: Front Panel State >> Open\nMacro: Interlock", "State(s) in (\"\")"=w332) -> ("States Out"=w331:string)  [unwired: 13 in]
      }
      frame "Macro: Interlock" {
        n116 = call <vilib>:"Add State(s) to Queue__JKI_lib_State_Machine.vi"("State(s) in Front (\"\")"="UI: Update Status\nUI: Update Interlock", "State(s) in (\"\")"=w338) -> ("States Out"=w337:string)  [unwired: 13 in]
      }
      frame "Macro: Load Sequence" {
        n117 = call <vilib>:"Add State(s) to Queue__JKI_lib_State_Machine.vi"("State(s) in Front (\"\")"="Sequence: Load\nData: Set Seq. Loaded Flag >> True\nOutgoing Messages: Status\nUI: Update MCL\nMacro: Interlock", "State(s) in (\"\")"=w344) -> ("States Out"=w343:string)  [unwired: 13 in]
      }
      frame "Macro: Run Sequence" {
        n118 = Unbundle By Name(w357) -> ("Running Step #"=w355:i32, "Sequence Data [ ]"=w356:T6[])
        n119 = Increment(x=w355) -> (x+1=w346:i32)
        n120 = Array Size(array=w356) -> (size(s)=w354:i32)
        n121 = Decrement(x=w354) -> (x-1=w351:i32)
        n122 = In Range and Coerce(upper limit=w351, x=w346, lower limit=0) -> (In Range?=w352:bool)  [unwired: 1 out]
        n123 = Format Into String(format string="Data: Set Running Step >> %d\nOutgoing Messages: Status\nMacro: Interlock\nMacro: Run Step\nMacro: Run Sequence ", w346) -> (resulting string=w349:string)  [unwired: 2 in, 1 out]
        n124 = Select(t=w349, s=w352, f="Data: Set Running Step >> -1\nOutgoing Messages: Status\nMacro: Interlock") -> (s? t:f=w347:string)
        n125 = call <vilib>:"Add State(s) to Queue__JKI_lib_State_Machine.vi"("State(s) in Front (\"\")"=w347, "State(s) in (\"\")"=w360) -> ("States Out"=w359:string)  [unwired: 13 in]
      }
      frame "Macro: Run Step" {
        # "Initialization Macro\n(This is called once, when the VI starts)"
        n126 = call <vilib>:"Add State(s) to Queue__JKI_lib_State_Machine.vi"("State(s) in Front (\"\")"="Sequence: Get Step\nIO: Write all DO\nIO: Write all AO\nIO: Dwell", "State(s) in (\"\")"=w366) -> ("States Out"=w365:string)  [unwired: 13 in]
      }
      frame "Macro: Abort Sequence" {
        n127 = call <vilib>:"Add State(s) to Queue__JKI_lib_State_Machine.vi"("State(s) in Front (\"\")"="Data: Set Seq. Aborted Flag >> True\nOutgoing Messages: Status\nMacro: Interlock\nIO: Dwell  // finish current step (remove to abort immediately)\nData: Set Running Step >> -1\nOutgoing Messages: Status\n// UI: Update Table Selection\nData: Set Seq. Aborted Flag >> False\nOutgoing Messages: Status\nMacro: Interlock") -> ("States Out"=w371:string)  [unwired: 14 in]
      }
      frame "Macro: Exit" {
        # "Exit Macro\n(This is called once, when the VI exits)"
        n128 = Unbundle By Name(w379) -> ("Core.Close Panel on Exit?"=w378:bool)
        n129 = Select(t="UI: Front Panel State >> Close", s=w378, f="") -> (s? t:f=w375:string)
        n130 = call <vilib>:"Add State(s) to Queue__JKI_lib_State_Machine.vi"("State(s) in (\"\")"=w375, "State(s) at Back (\"\")"="Data: Cleanup\nEvents: Unregister\nExit") -> ("States Out"=w373:string)  [unwired: 13 in]
        n131 = call <vilib>:"Add State(s) to Queue__JKI_lib_State_Machine.vi"("State(s) in Front (\"\")"=w373, "State(s) in (\"\")"=w382) -> ("States Out"=w381:string)  [unwired: 13 in]
      }
      frame "---------- IO ----------" {
        # "Template Separator\n(You can make a copy of, or modify, this frame)"
        n132 = call <vilib>:"Add State(s) to Queue__JKI_lib_State_Machine.vi"("State(s) in (\"\")"=w387) -> ("States Out"=w386:string)  [unwired: 14 in]
      }
      frame "IO: Write all DO" {
        n133 = Unbundle By Name(w390) -> ("DO Data [ ]"=w389:cluster{"DO Name":string, "DO Value":variant}[])
        n134 = call "DO.Write.vi"("error in (no error)"=w392, "DO Data"=w389) -> ("error out"=w391:errorcluster)  [unwired: 9 in]
        n135 = call <vilib>:"Add State(s) to Queue__JKI_lib_State_Machine.vi"("State(s) in (\"\")"=w394) -> ("States Out"=w393:string)  [unwired: 14 in]
      }
      frame "IO: Write all AO" {
        n136 = Unbundle By Name(w399) -> ("AO Data [ ]"=w398:cluster{"AO Name":string, "AO Value":variant}[])
        n137 = call "AO.Write.vi"("error in (no error)"=w397, "AO Data"=w398) -> ("error out"=w396:errorcluster)  [unwired: 9 in]
        n138 = call <vilib>:"Add State(s) to Queue__JKI_lib_State_Machine.vi"("State(s) in (\"\")"=w401) -> ("States Out"=w400:string)  [unwired: 14 in]
      }
      frame "IO: Dwell" {
        n139 = Unbundle By Name(w414) -> ("Sequence Data [ ]"=w418:T6[], "Running Step #"=w417:i32, "Seq. Aborted?"=w405:bool)
        n140 = Index Array(array=w418, index=w417) -> (element=w416:T6)
        n141 = Unbundle By Name(w416) -> ("Dwell Time(s)"=w415:dbl)
        n142 = call <userlib>:"Boolean Trigger__ogtk.vi"("Boolean Input"=w405) -> ("Falling Edge"=w408:bool)  [unwired: 1 in, 1 out]
        n143 = expression code="x*1000"(w415) -> (w404:dbl)
        n144 = feedback #1() -> (w407:bool)  [unwired: 1 in]
        n145 = Or(x=w407, y=w408) -> (x .or. y?=w406:bool)
        n146 = call <userlib>:"Periodic Trigger__ogtk.vi"("time (ms)"=w404, "reset"=w406) -> ("Triggered"=w409:bool, "timer value"=→"timer value":u32)  [unwired: 11 in, 1 out]
        n147 = feedback-in #1(w409) -> ()
        n148 = Select(t="", s=w409, f="Idle  //Calls event structure\nIO: Dwell //Come back Here") -> (s? t:f=w403:string)
        n149 = call <vilib>:"Add State(s) to Queue__JKI_lib_State_Machine.vi"("State(s) in Front (\"\")"=w403, "State(s) in (\"\")"=w420) -> ("States Out"=w419:string)  [unwired: 13 in]
      }
      frame "---------- Sequence ----------" {
        # "Template Separator\n(You can make a copy of, or modify, this frame)"
        n150 = call <vilib>:"Add State(s) to Queue__JKI_lib_State_Machine.vi"("State(s) in (\"\")"=w425) -> ("States Out"=w424:string)  [unwired: 14 in]
      }
      frame "Sequence: Load" {
        # "Valid Path\nAND\nNot a Directory\nAND\nExist"
        n151 = Unbundle By Name(w435) -> ("Sequence file path"=w431:path)
        n152 = call-poly <userlib>:"Valid Path__ogtk.vi"("path"=w431) -> ("valid"=w432:bool)
        n153 = call-poly <userlib>:"File Exists__ogtk.vi"("file path"=w431) -> ("is directory"=w433:bool, "exists"=w434:bool)  [unwired: 6 in]
        n154 = Compound Arithmetic op=AND(w432, invert w433, w434) -> (w427:bool)
        n155 = case "\"Good\" sequence file path?" shown="True" w427 {
          tunnel: w431 -> [_ w445]
          tunnel: w430 -> [w441 w444]
          tunnel: [w440 w443] -> w429
          tunnel: [w439 w442] -> w428
          frame False {
            # "No, then ask user to select one"
            n156 = call "Sequence.Load.vi"("error in (no error)"=w441) -> ("error out"=w440:errorcluster, "Sequence Data [ ]"=w439:T6[])  [unwired: 8 in, 1 out]
          }
          frame True {
            # "Yes, then load it"
            n157 = call "Sequence.Read.vi"("error in (no error)"=w444, "Recipe file path"=w445) -> ("error out"=w443:errorcluster, "Recipe Data"=w442:T6[])  [unwired: 7 in, 1 out]
          }
        }
        n158 = Bundle By Name(cluster=w435, "Sequence Data [ ]"=w428) -> (w436:T9)
        n159 = call <vilib>:"Add State(s) to Queue__JKI_lib_State_Machine.vi"("State(s) in (\"\")"=w438) -> ("States Out"=w437:string)  [unwired: 14 in]
      }
      frame "Sequence: Get Step" {
        n160 = Unbundle By Name(w451) -> ("Sequence Data [ ]"=w450:T6[], "Running Step #"=w449:i32)
        n161 = call "Sequence.GetStep.vi"("error in (no error)"=w453, "Step #"=w449, "Sequence Data"=w450) -> ("error out"=w452:errorcluster, "AO [ ]"=w447:cluster{"IO Name":string, "IO Value":variant}[], "DO [ ]"=w448:cluster{"IO Name":string, "IO Value":variant}[])  [unwired: 6 in]
        n162 = Bundle By Name(cluster=w451, "DO Data [ ]"=w448, "AO Data [ ]"=w447) -> (w454:T9)
        n163 = call <vilib>:"Add State(s) to Queue__JKI_lib_State_Machine.vi"("State(s) in (\"\")"=w456) -> ("States Out"=w455:string)  [unwired: 14 in]
      }
      frame "---------- Outgoing Messages ----------" {
        # "Template Separator\n(You can make a copy of, or modify, this frame)"
        n164 = call <vilib>:"Add State(s) to Queue__JKI_lib_State_Machine.vi"("State(s) in (\"\")"=w461) -> ("States Out"=w460:string)  [unwired: 14 in]
      }
      frame "Outgoing Messages: Status" {
        # "Valid?"
        n165 = Unbundle By Name(w471) -> ("Outbound User Events.Sequencer Status"=w464:refnum<user-event>, "Seq. Loaded?"=w468:bool, "Seq. Running?"=w470:bool, "Seq. Aborted?"=w469:bool)
        n166 = Bundle("Seq. Loaded?"=w468, "Seq. Running?"=w470, "Seq. Aborted?"=w469) -> (w467:T11)  [unwired: 1 in]
        n167 = Not A Number/Path/Refnum?(number/path/refnum=w464) -> (NaN/Path/Refnum?=w463:bool)
        n168 = Not(x=w463) -> (.not. x?=w462:bool)
        n169 = case shown="True" w462 {
          tunnel: w467 -> [_ w479]
          tunnel: [w475 w478] -> w466
          tunnel: w465 -> [w475 w477]
          tunnel: w464 -> [_ w476]
          frame False {
          }
          frame True {
            n170 = Generate User Event(user event=w476, event data cluster=w479, error in=w477) -> (error out=w478:errorcluster)  [unwired: 1 in, 1 out]
          }
        }
        n171 = call <vilib>:"Add State(s) to Queue__JKI_lib_State_Machine.vi"("State(s) in (\"\")"=w474) -> ("States Out"=w473:string)  [unwired: 14 in]
      }
      frame "Outgoing Messages: AO Data" {
        # "Valid?"
        n172 = Unbundle By Name(w483) -> ("Outbound User Events.AO Data"=w484:refnum<user-event>, "Sequence Data [ ]"=w487:T6[], "Running Step #"=w486:i32)
        n173 = call "Sequence.GetStep.vi"("error in (no error)"=w480, "Step #"=w486, "Sequence Data"=w487) -> ("error out"=w485:errorcluster, "AO [ ]"=w488:cluster{"IO Name":string, "IO Value":variant}[])  [unwired: 6 in, 1 out]
        n174 = Not A Number/Path/Refnum?(number/path/refnum=w484) -> (NaN/Path/Refnum?=w490:bool)
        n175 = call "Graph.UpdateAOs.vi"("error in (no error)"=w485, "AO Data [ ]"=w488) -> ("error out"=w481:errorcluster, "Graph Data"=w482:cluster{"[0]":dbl, "[1]":dbl})  [unwired: 8 in]
        n176 = Not(x=w490) -> (.not. x?=w489:bool)
        n177 = case shown="True" w489 {
          tunnel: w482 -> [_ w499]
          tunnel: [w495 w498] -> w491
          tunnel: w481 -> [w495 w497]
          tunnel: w484 -> [_ w496]
          frame False {
          }
          frame True {
            n178 = Generate User Event(user event=w496, event data cluster=w499, error in=w497) -> (error out=w498:errorcluster)  [unwired: 1 in, 1 out]
          }
        }
        n179 = call <vilib>:"Add State(s) to Queue__JKI_lib_State_Machine.vi"("State(s) in (\"\")"=w494) -> ("States Out"=w493:string)  [unwired: 14 in]
      }
    }
  }
  n180 = disable-structure shown="Disabled" {
    frame Disabled {
      n181 = flat-sequence "IO Utilities" {
        frame #0 {
        }
      }
      n182 = flat-sequence "Sequence Utilities" {
        frame #0 {
        }
      }
    }
    frame Enabled {
    }
  }
